vi "_ConvertResTable.vi"(0 "ResTable":dbl[][](array[numeric]) format="%.2f") -> (1 "HiResTable":dbl[][](array[numeric]), 2 "MidResTable":dbl[][](array[numeric]), 3 "LowResTable":dbl[][](array[numeric]))   [LabVIEW 2015]
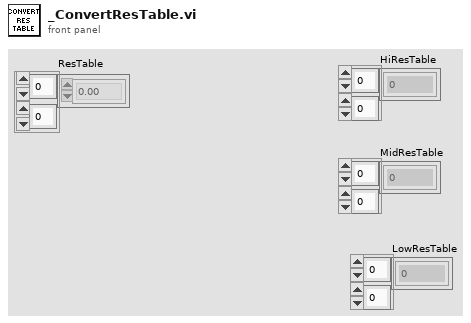
[diagram p1: front panel]
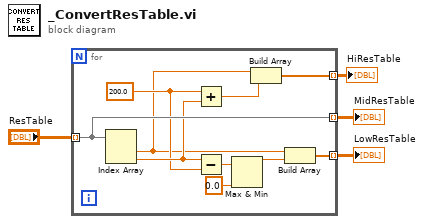
[diagram p0: block diagram]
diagram:
  n1 = for {
    tunnel: "ResTable" -> [w14] mode=indexing
    tunnel: [w14] -> w1 mode=indexing
    tunnel: [w8] -> w3 mode=indexing
    tunnel: [w5] -> w2 mode=indexing
    w12 = 200.0 ("x")
    n2 = Index Array(array=w14) -> (element #1=w6:dbl, element #2=w13:dbl)  [unwired: 2 in]
    n3 = Add(x=w12, y=w13) -> (x+y=w9:dbl)
    n4 = Subtract(x=w13, y=w12) -> (x-y=w11:dbl)
    n5 = Max & Min(x=w11, y=0.0) -> (max(x,y)=w7:dbl)  [unwired: 1 out]
    n6 = Build Array(w6, w9) -> (w8:dbl[])
    n7 = Build Array(w6, w7) -> (w5:dbl[])
  }
  "HiResTable" <- w3
  "MidResTable" <- w1
  "LowResTable" <- w2
